vi "send on connection.vi"(8 "error in":errorcluster, 9 "timeout ms (10000)":i32=10000, 10 "data message":refnum<class "communicator message.lvclass">, 11 "connection in":refnum<class "Queue connection.lvclass">) -> (0 "error out":errorcluster, 3 "connection out":refnum<class "Queue connection.lvclass">)   [LabVIEW 2015, in "Queue connection.lvclass"]
uses:
  Queue connection.lvclass
  message/communicator message.lvclass
  Queue connection.lvclass/Queue connection.ctl
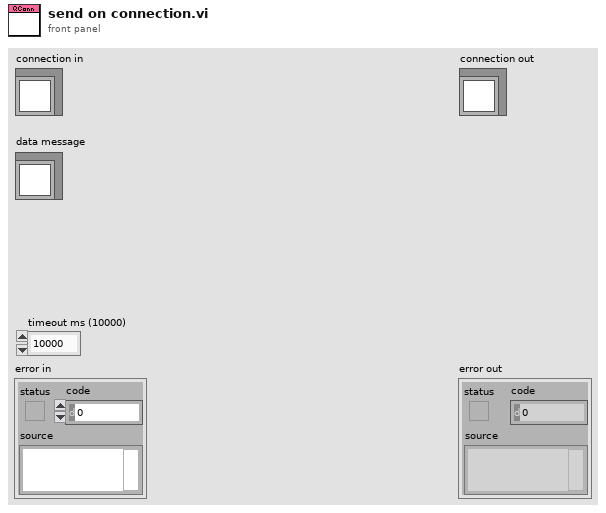
[diagram p1: front panel]
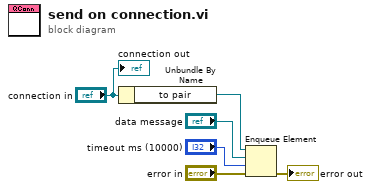
[diagram p0: block diagram]
diagram:
  n1 = Unbundle By Name("connection in") -> ("to pair"=w3:refnum<queue>)
  n2 = Enqueue Element(queue=w3, element="data message", timeout in ms (-1)="timeout ms (10000)", error in (no error)="error in") -> (error out=→"error out":errorcluster)  [unwired: 2 out]
  "connection out" <- "connection in"
